vi "BASE_I_O_Manual.vi"(8 "error in (no error)":errorcluster) -> (0 "error out":errorcluster)   [LabVIEW 2017]
doc: "This vi is for manually turn ON and OFF also monitor Output of PLCS. So this is manual screen."
uses:
  Global/PLC_to_Auto.vi
panel:
  in  "Tab Control":enum32{"MANUAL SWITCH", "SCANNER"}(tab)
  in  "PART DECLAMP SOL":bool
  in  "PART CLAMP SOL":bool
  in  "THREAD LOCKER ON":bool
  in  "THREAD LOCKER OFF":bool
  in  "PUSHER FWD SOL":bool
  in  "PUSHER REV SOL":bool
  in  "THREAD LOCKER CYL DOWN ON":bool
  in  "THREAD LOCKER CYL UP ON":bool
  in  "AUTO/MANUAL":bool
  in  "Flush Scaner":bool
  out "SCANNED STRING":string
  in  "Leght of byte to read":bool
  in  "scan":bool
  out "SCANNED COM PORT":refnum<visa-resource-name>
  out "error out 3":errorcluster
  out "error out 4":errorcluster
  in  "Back":bool
  # "BARCODE VERIFICATION SYSTEM REPORTS"
  # "Manual Cycle"
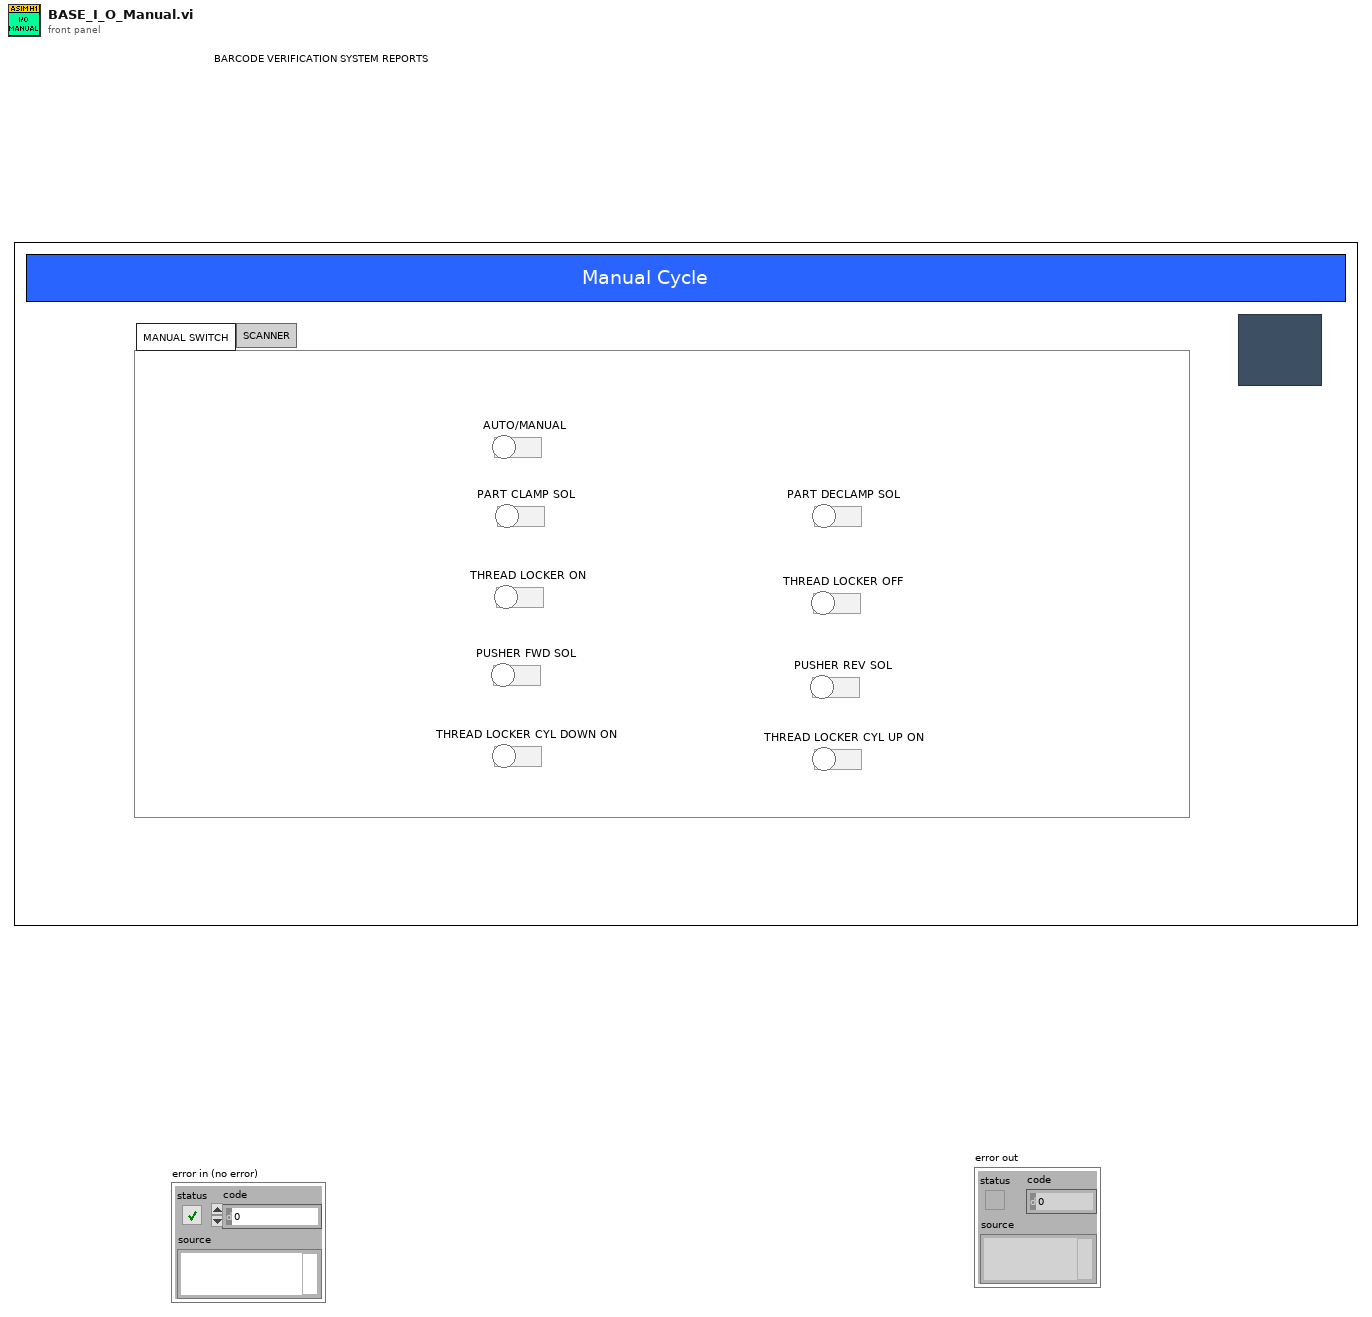
[diagram p1: front panel]
types:
  T1 = cluster{"IP Address":string, "LH Scanner IP Address":string, "RH Scanner IP Address":string}
  T2 = enum32{"invalid app kind", "Development System", "Run Time System", "Student Edition", "Embedded LabVIEW", "Evaluation", "Custom"}
  T3 = enum32{"Invalid", "Standard", "Closed", "Hidden", "Minimized", "Maximized"}
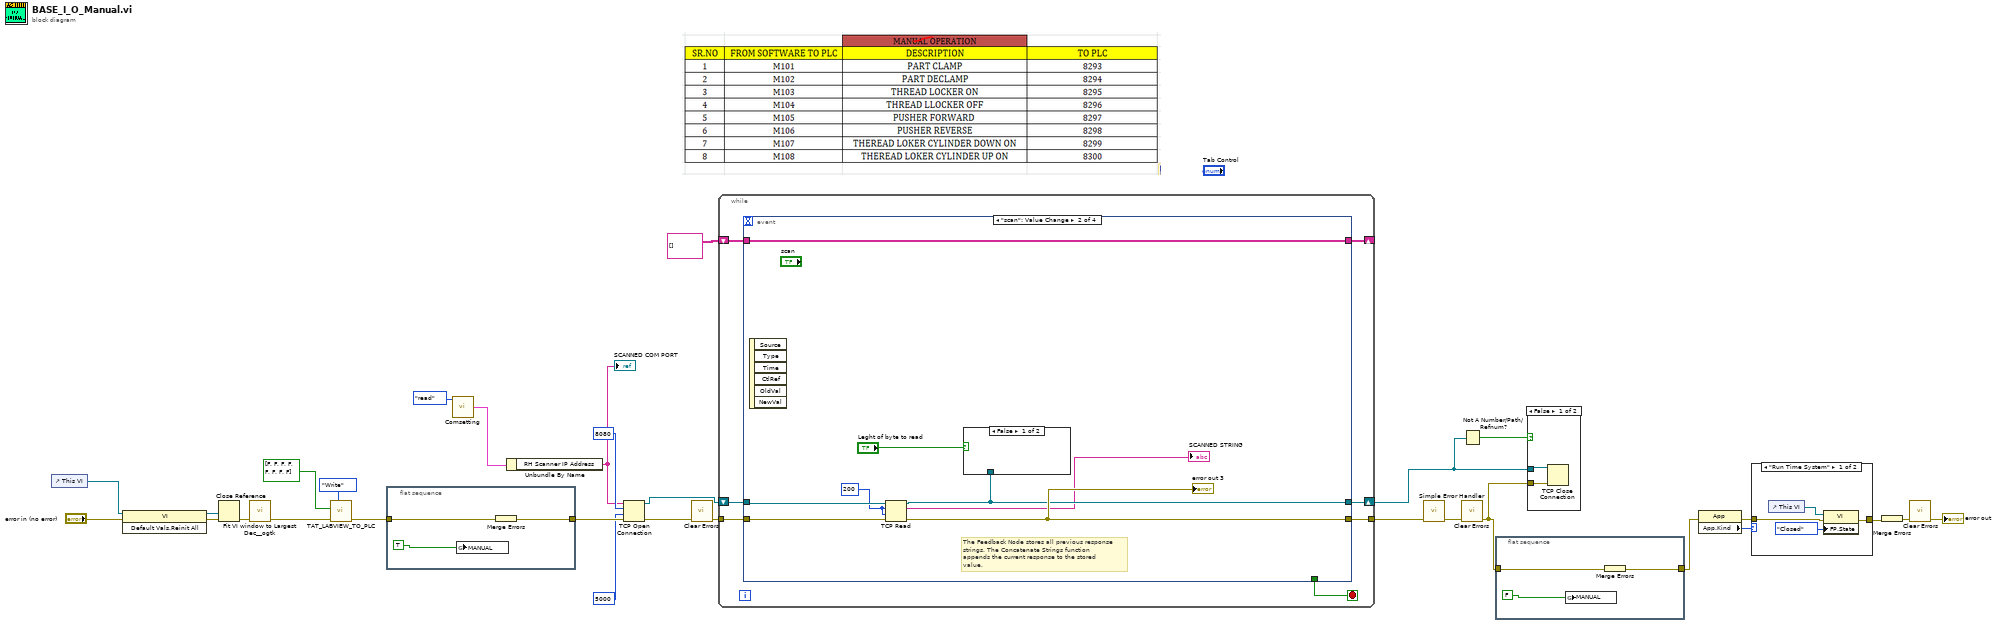
[diagram p0: block diagram]
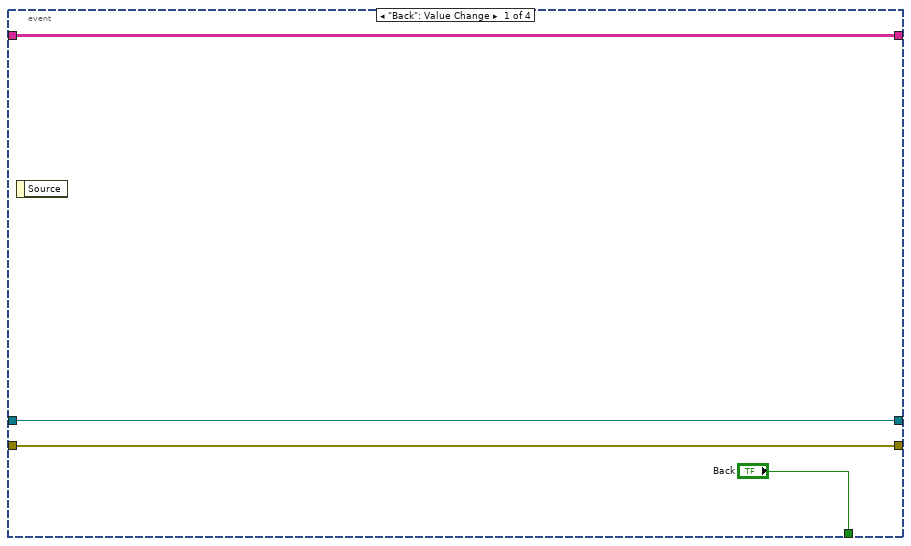
[diagram p4: hidden frame]
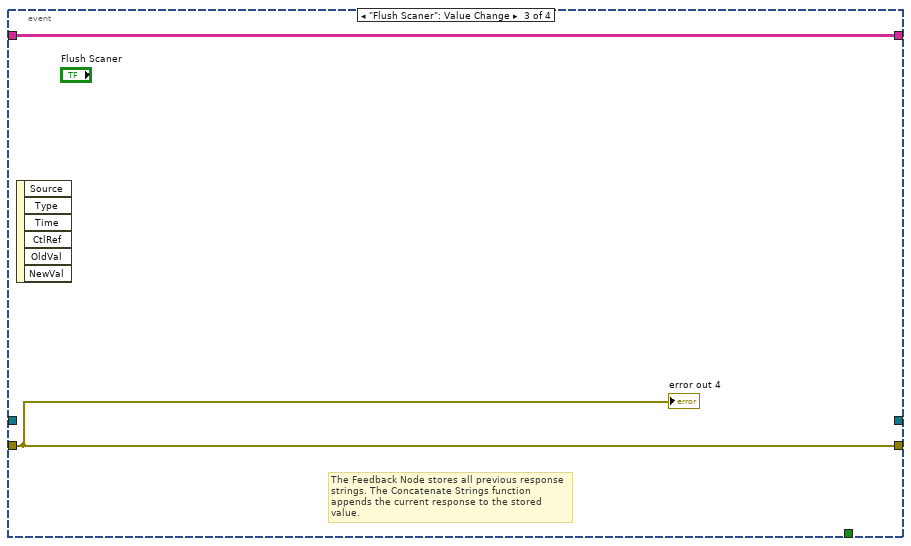
[diagram p6: hidden frame]
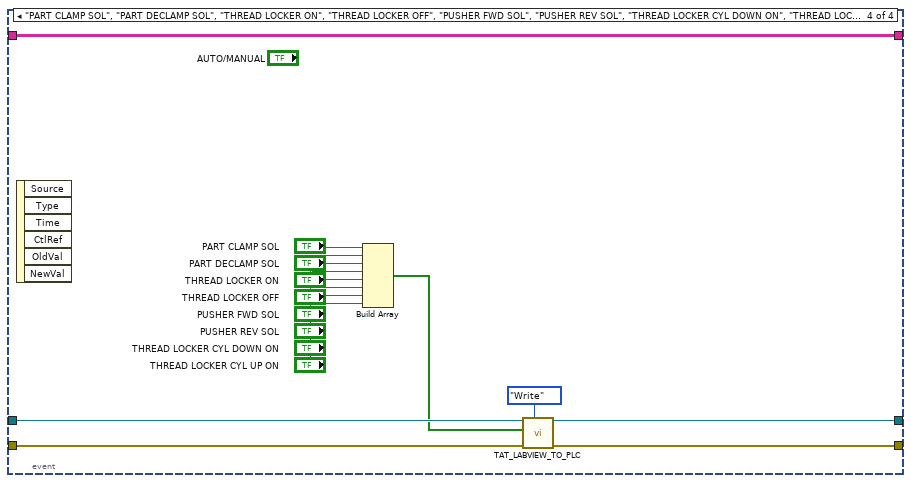
[diagram p7: hidden frame]
diagram:
  n1 = control-ref of="This VI"() -> (w25:refnum<vi>)
  n2 = invoke class="VI" method="Default Vals.Reinit All"(reference=w25, error in="error in (no error)") -> (reference out=w23:refnum<vi>, error out=w22:errorcluster)  [unwired: 1 in, 1 out]
  n3 = Close Reference(reference=w23, error in (no error)=w22) -> (error out=w21:errorcluster)
  n4 = call <userlib>:"Fit VI window to Largest Dec__ogtk.vi"("error in (no error)"=w21) -> ("error out"=w11:errorcluster)  [unwired: 5 in, 1 out]
  n5 = call "TAT_LABVIEW_TO_PLC.vi"("Enum"=enum16{"Read", "Write"}."Write", "error in (no error)"=w11, "Array"=bool[] [FALSE, FALSE, FALSE, FALSE, FALSE, FALSE, FALSE, FALSE]) -> ("error out"=w10:errorcluster)  [unwired: 7 in, 1 out]
  n6 = flat-sequence {
    tunnel: w10 -> [w33]
    tunnel: [w32] -> w15
    frame #0 {
      n7 = global write "PLC_to_Auto.vi" "MANUAL"(TRUE) -> ()
      n8 = Merge Errors(w33) -> (w32:errorcluster)
    }
  }
  n9 = call "Comsetting.vi"("Enum"=enum16{"read", "write"}."read") -> ("Cluster Out"=w16:T1)  [unwired: 2 in, 2 out]
  n10 = Unbundle By Name(w16) -> ("RH Scanner IP Address"=w3:string)
  "SCANNED COM PORT" <- w3
  n11 = TCP Open Connection(address=w3, remote port or service name=u16 8080, timeout ms (60000)=5000, error in (no error)=w15) -> (connection ID=w2:refnum<k5>, error out=w5:errorcluster)  [unwired: 1 in]
  n12 = call <vilib>:"Clear Errors.vi"("error in (no error)"=w5) -> ("error out"=w6:errorcluster)  [unwired: 5 in, 1 out]
  n13 = while {
    tunnel: w6 -> [w40]
    tunnel: [w39] -> w29
    shift-right: [w37] -> _
    shift-left: string[][] [] -> [w36]
    shift-right: [w34] -> w7
    shift-left: w2 -> [w35]
    stop <- w38 stop-if-true
    n14 = event shown="[1] \"scan\": Value Change" {
      selector: _ -> [_ _ _ _]
      dyn-events: _ -> [_ _ _ _]
      timeout: _ -> [_ _ _ _]
      tunnel: w40 -> [w43 w51 w53 w56]
      tunnel: [w43 w49 w53 w55] -> w39
      tunnel: ["Back" _ _ _] -> w38
      tunnel: [w42 w52 w54 w67] -> w37
      tunnel: w36 -> [w42 w52 w54 w67]
      tunnel: w35 -> [w41 w48 _ w68]
      tunnel: [w41 w47 _ w68] -> w34
      event "Back": Value Change {
        n15 = event-data() -> ()  [unwired: 1 in, 1 out]
      }
      event "scan": Value Change {
        w45 = 200 ("bytes to read")
        # "The Feedback Node stores all previous response strings. The Concatenate Strings function appends the current response to the stored value."
        n16 = event-data() -> ()  [unwired: 1 in, 6 out]
        n17 = TCP Read(connection ID=w48, bytes to read=w45, error in (no error)=w51, 9:w45) -> (connection ID out=w47:refnum<k5>, data out=→"SCANNED STRING":string, error out=w49:errorcluster)  [unwired: 1 in]
        "error out 3" <- w49
        n18 = case shown="False" "Leght of byte to read" {
          tunnel: w47 -> [_ _]
          frame False {
          }
          frame True {
          }
        }
      }
      event "Flush Scaner": Value Change {
        # "The Feedback Node stores all previous response strings. The Concatenate Strings function appends the current response to the stored value."
        n19 = event-data() -> ()  [unwired: 1 in, 6 out]
        "error out 4" <- w53
      }
      event "PART CLAMP SOL", "PART DECLAMP SOL", "THREAD LOCKER ON", "THREAD LOCKER OFF", "PUSHER FWD SOL", "PUSHER REV SOL", "THREAD LOCKER CYL DOWN ON", "THREAD LOCKER CYL UP ON", "AUTO/MANUAL": Value Change {
        n20 = event-data() -> ()  [unwired: 1 in, 6 out]
        n21 = Build Array("PART CLAMP SOL", "PART DECLAMP SOL", "THREAD LOCKER ON", "THREAD LOCKER OFF", "PUSHER FWD SOL", "PUSHER REV SOL", "THREAD LOCKER CYL DOWN ON", "THREAD LOCKER CYL UP ON") -> (w57:bool[])
        n22 = call "TAT_LABVIEW_TO_PLC.vi"("Enum"=enum16{"Read", "Write"}."Write", "error in (no error)"=w56, "Array"=w57) -> ("error out"=w55:errorcluster)  [unwired: 7 in, 1 out]
      }
    }
  }
  n23 = call <vilib>:"Simple Error Handler.vi"("error in (no error)"=w29) -> ("error out"=w20:errorcluster)  [unwired: 4 in, 4 out]
  n24 = call <vilib>:"Clear Errors.vi"("error in (no error)"=w20) -> ("error out"=w14:errorcluster)  [unwired: 5 in, 1 out]
  n25 = Not A Number/Path/Refnum?(number/path/refnum=w7) -> (NaN/Path/Refnum?=w8:bool)
  n26 = flat-sequence {
    tunnel: w14 -> [w71]
    tunnel: [w70] -> w13
    frame #0 {
      n27 = global write "PLC_to_Auto.vi" "MANUAL"(FALSE) -> ()
      n28 = Merge Errors(w71) -> (w70:errorcluster)
    }
  }
  n29 = case shown="False" w8 {
    tunnel: w7 -> [w72 _]
    tunnel: w14 -> [w73 _]
    frame False {
      n30 = TCP Close Connection(connection ID=w72, error in (no error)=w73) -> ()  [unwired: 1 in, 2 out]
    }
    frame True {
    }
  }
  n31 = property class="App"(error in=w13) -> (error out=w18:errorcluster, "App.Kind"=w19:T2)  [unwired: 1 in, 1 out]
  n32 = case shown="\"Run Time System\"" w19 {
    tunnel: w18 -> [w75 w78]
    tunnel: [w74 w78] -> w27
    frame "Run Time System" {
      n33 = control-ref of="This VI"() -> (w77:refnum<vi>)
      n34 = property class="VI"(reference=w77, error in=w75, "FP.State"=T3."Closed" ("Front Panel Window:State")) -> (error out=w74:errorcluster)  [unwired: 1 out]
    }
    frame "Development System", Default {
    }
  }
  n35 = Merge Errors(w27) -> (w28:errorcluster)
  n36 = call <vilib>:"Clear Errors.vi"("error in (no error)"=w28) -> ("error out"=→"error out":errorcluster)  [unwired: 5 in, 1 out]
